vi "Math part.vi"() -> ()   [LabVIEW 2020]
panel:
  out "SDO":u64[](array[numeric]) format="%.0x"
  out "max(x,y)":i32[](array[numeric])
  out "x*y":i32
  in  "SDI":u64[](array[numeric]) format="%.0x"
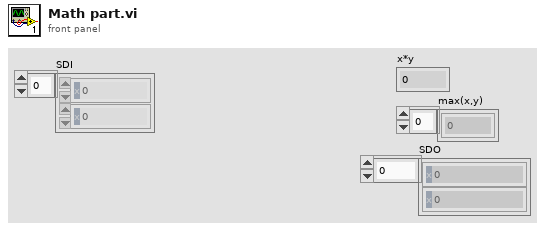
[diagram p1: front panel]
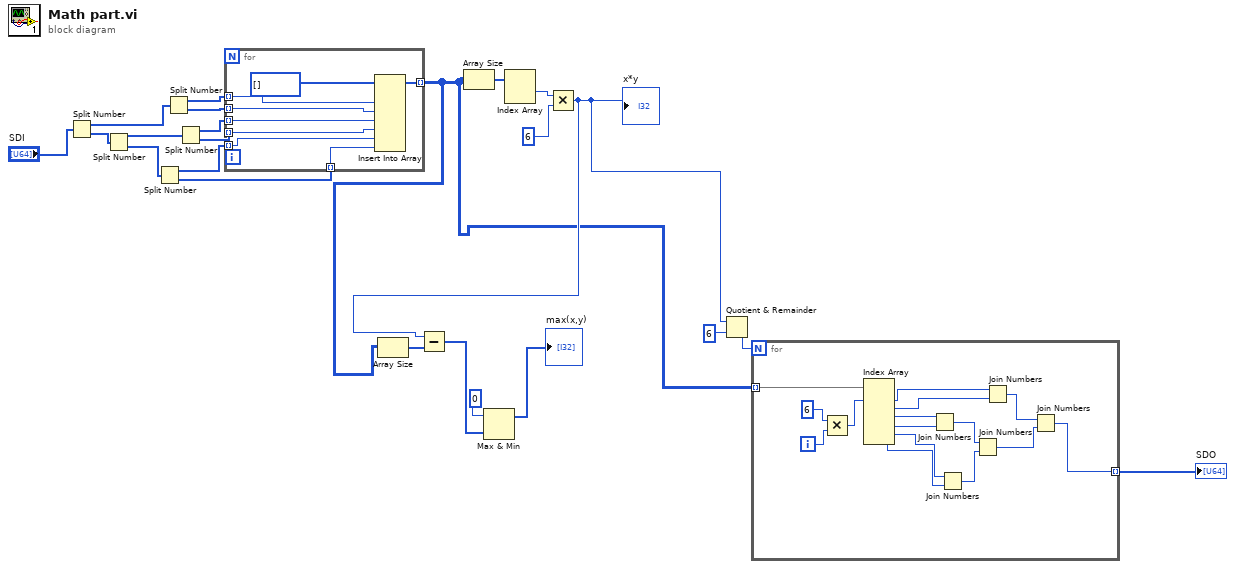
[diagram p0: block diagram]
diagram:
  n1 = Split Number(x="SDI") -> (hi(x)=w22:u32[], lo(x)=w3:u32[])
  n2 = Split Number(x=w3) -> (hi(x)=w5:u16[], lo(x)=w4:u16[])
  n3 = Split Number(x=w4) -> (hi(x)=w2:u8[], lo(x)=w1:u8[])
  n4 = Split Number(x=w22) -> (hi(x)=w21:u16[], lo(x)=w20:u16[])
  n5 = Split Number(x=w5) -> (hi(x)=w19:u8[], lo(x)=w18:u8[])
  n6 = for {
    tunnel: w21 -> [w31] mode=indexing
    tunnel: w20 -> [w26] mode=indexing
    tunnel: w19 -> [w30] mode=indexing
    tunnel: w18 -> [w29] mode=indexing
    tunnel: [w28] -> w7 mode=indexing
    tunnel: w2 -> [w25] mode=indexing
    tunnel: w1 -> [w24] mode=indexing
    n7 = Insert Into Array(array=u8[] [], new element #1=w31, new element #2=w26, new element #3=w30, new element #4=w29, new element #5=w25, new element #6=w24) -> (w28:u8[])  [unwired: 1 in]
  }
  n8 = Array Size(array=w7) -> (size(s)=w13:i32[])
  n9 = Array Size(array=w7) -> (size(s)=w23:i32[])
  n10 = Index Array(array=w23) -> (element #1=w12:i32)  [unwired: 2 in, 1 out]
  n11 = Multiply(x=w12, y=6) -> (x*y=w9:i32)
  "x*y" <- w9
  n12 = Subtract(x=w9, y=w13) -> (x-y=w16:i32[])
  n13 = Max & Min(x=0, y=w16) -> (max(x,y)=→"max(x,y)":i32[])  [unwired: 1 out]
  n14 = Quotient & Remainder(x=w9, y=6) -> (floor(x/y)=w10:i32)  [unwired: 1 out]
  n15 = for {
    N: w10 -> [_]
    tunnel: [w41] -> w8 mode=indexing
    tunnel: w7 -> [w39] mode=indexing
    i -> [w40]
    n16 = Multiply(x=6, y=w40) -> (x*y=w45:i32)
    n17 = Index Array(array=w39, index #1=w45) -> (element #1=w44:u8, element #2=w42:u8, element #3=w38:u8, element #4=w37:u8, element #5=w36:u8, element #6=w35:u8)  [unwired: 5 in]
    n18 = Join Numbers(hi=w38, lo=w37) -> ((hi.lo)=w34:u16)
    n19 = Join Numbers(hi=w36, lo=w35) -> ((hi.lo)=w33:u16)
    n20 = Join Numbers(hi=w34, lo=w33) -> ((hi.lo)=w32:u32)
    n21 = Join Numbers(hi=w44, lo=w42) -> ((hi.lo)=w43:u16)
    n22 = Join Numbers(hi=w43, lo=w32) -> ((hi.lo)=w41:u64)
  }
  "SDO" <- w8
